vi "Create.vi"   [LabVIEW 2018, in "Toolkit.lvlib" / "Known Host.lvclass"]
uses:
  Known Host.lvclass
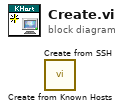
[diagram p0: block diagram]
diagram:
  n1 = call "Create from Known Hosts.vi"() -> ()  [unwired: 9 in, 3 out]
  n2 = call "Create from SSH.vi"() -> ()  [unwired: 10 in, 2 out]
